vi "Write One-Port Cal Standards.vi"(8 "error in (no error)":errorcluster, 10 "One-Port Cal Standards":T1[](array[typedef]), 11 "Cal Standard Base in":refnum<class "Cal Standard Base.lvclass">) -> (0 "error out":errorcluster, 3 "Cal Standard Base out":refnum<class "Cal Standard Base.lvclass">)   [LabVIEW 2023, in "RFFixtureCharact.Instruments.lvlib" / "Cal Standard Base.lvclass"]
uses:
  Cal Standard Base.lvclass
  Type Definitions/One-Port Cal Standard.ctl
  Type Definitions/One-Port Charact Data.ctl
  Type Definitions/Standard Type.ctl
  Cal Standard Base.lvclass/Cal Standard Base.ctl
  RFFixtureCharact.Instruments.lvlib
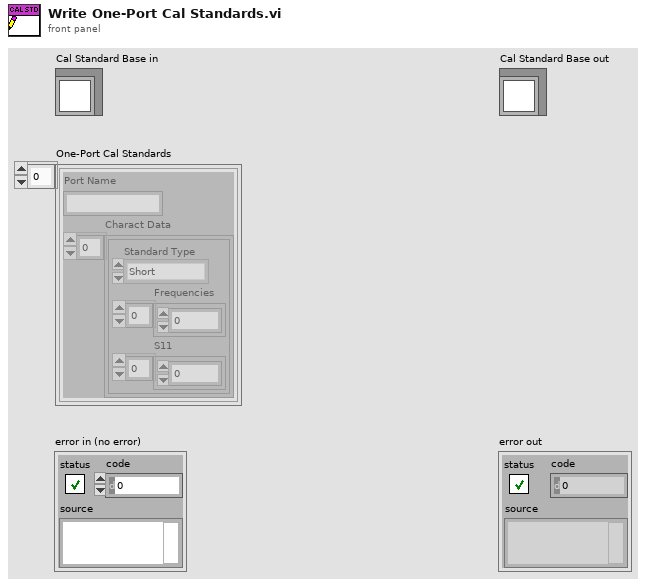
[diagram p1: front panel]
types:
  T1 = typedef "RFFixtureCharact.Instruments.lvlib/One-Port Cal Standard.ctl" = cluster{"Port Name":string, "Charact Data":T2[]}
  T2 = typedef "RFFixtureCharact.Instruments.lvlib/One-Port Charact Data.ctl" = cluster{"Standard Type":T3, "Frequencies":dbl[], "S11":cdb[]}
  T3 = typedef "RFFixtureCharact.Instruments.lvlib/Standard Type.ctl" = enum16{"Short", "Open", "Load"}
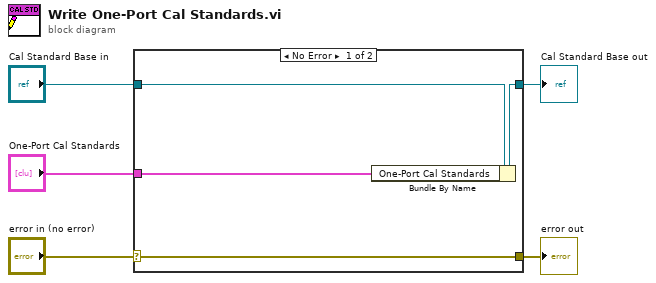
[diagram p0: block diagram]
diagram:
  n1 = case shown="No Error" "error in (no error)" {
    selector: "error in (no error)" -> [w9 w10]
    tunnel: [w9 w10] -> w4
    tunnel: [w7 w11] -> w2
    tunnel: "Cal Standard Base in" -> [w8 w11]
    tunnel: "One-Port Cal Standards" -> [w6 _]
    frame No Error {
      n2 = Bundle By Name(cluster=w8, "One-Port Cal Standards"=w6) -> (w7:refnum<class "Cal Standard Base.lvclass">)
    }
    frame Error {
    }
  }
  "error out" <- w4
  "Cal Standard Base out" <- w2
